vi "checkin.vi"(8 "error in (no error)":errorcluster, 11 "GenericPlugin in":refnum<class "GenericToplevelComponent.lvclass">) -> (0 "error out":errorcluster, 3 "GenericPlugin out":refnum<class "GenericToplevelComponent.lvclass">)   [LabVIEW 2010, in "GenericToplevelComponent.lvclass"]
uses:
  GenericToplevelComponent.lvclass
  enumerations/error_codes.ctl
  GenericComponent/GenericComponent/GenericComponent.lvclass
  GenericToplevelComponent.lvclass/GenericToplevelComponent.ctl
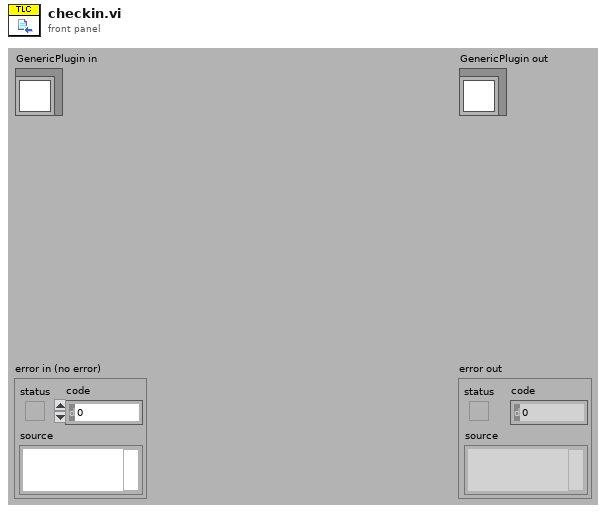
[diagram p1: front panel]
types:
  T1 = typedef "error_codes.ctl" = u16
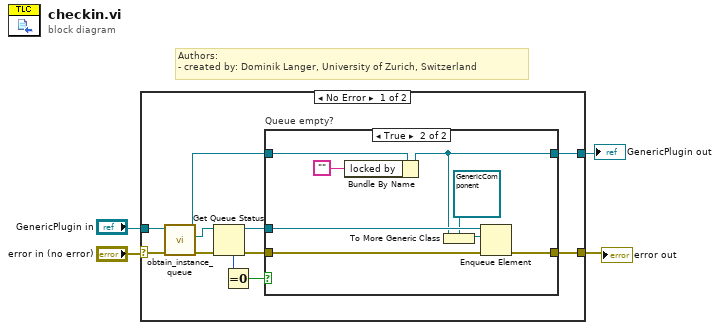
[diagram p0: block diagram]
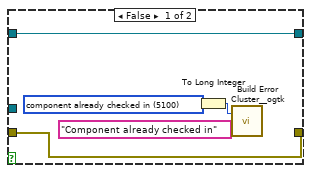
[diagram p2: hidden frame]
diagram:
  # "Authors: \n- created by: Dominik Langer, University of Zurich, Switzerland"
  n1 = case shown="No Error" "error in (no error)" {
    selector: "error in (no error)" -> [w10 w30]
    tunnel: [w12 w30] -> w2
    tunnel: [w11 w29] -> w1
    tunnel: "GenericPlugin in" -> [w8 w29]
    frame No Error {
      n2 = call-dynamic "obtain_instance_queue.vi"("error in (no error)"=w10, "GenericToplevelComponent in"=w8) -> ("error out"=w9:errorcluster, "instance queue"=w6:refnum<queue>, "GenericToplevelComponent out"=w7:refnum<class "GenericToplevelComponent.lvclass">)  [unwired: 7 in]
      n3 = Get Queue Status(queue=w6, error in (no error)=w9) -> (queue out=w5:refnum<queue>, error out=w15:errorcluster, # elements in queue=w13:i32)  [unwired: 6 out]
      n4 = Equal To 0?(x=w13) -> (x = 0?=w14:bool)
      n5 = case "Queue empty?" shown="True" w14 {
        tunnel: w15 -> [w16 w28]
        tunnel: [w16 w24] -> w12
        tunnel: w5 -> [_ w27]
        tunnel: w7 -> [w17 w26]
        tunnel: [w17 w23] -> w11
        frame False {
          w19 = T1 5100 items=["You can't check in if it is already checked in."=0, "component already checked in"=5100] ("Ring")
          n6 = To Long Integer(number=w19) -> (32bit integer=w18:i32)
          n7 = call <userlib>:"Build Error Cluster__ogtk.vi"("String to Prepend to source (\"\")"="Component already checked in" ("String to Prepend to source (\"\")"), "code"=w18) -> ()  [unwired: 1 out]
        }
        frame True {
          n8 = Bundle By Name(cluster=w26, "locked by"="") -> (w23:refnum<class "GenericToplevelComponent.lvclass">)
          n9 = To More Generic Class(target class=refnum<class "GenericComponent.lvclass"> refnum ("GenericComponent.lvclass"), reference=w23) -> (generic class reference=w22:refnum<class "GenericComponent.lvclass">)
          n10 = Enqueue Element(queue=w27, element=w22, error in (no error)=w28) -> (error out=w24:errorcluster)  [unwired: 3 out]
        }
      }
    }
    frame Error {
    }
  }
  "error out" <- w2
  "GenericPlugin out" <- w1
